vi "Write Name.vi"(10 "Name":string, 11 "Log Sink in":refnum<class "Log Sink.lvclass">) -> (3 "Log Sink out":refnum<class "Log Sink.lvclass">)   [LabVIEW 2017, in "Composed Log.lvlib" / "Log Sink.lvclass"]
uses:
  <vilib>/gpm_packages/@cs/event-logger/Source/Composed Log/Log Sink/Log Sink.lvclass
  <vilib>/gpm_packages/@cs/event-logger/Source/Composed Log/Log Sink/Log Sink.lvclass/Log Sink.ctl
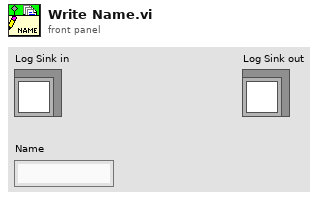
[diagram p1: front panel]
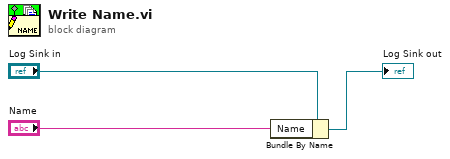
[diagram p0: block diagram]
diagram:
  n1 = Bundle By Name(cluster="Log Sink in", "Name"="Name") -> (→"Log Sink out":refnum<class "Log Sink.lvclass">)
